vi "Use FGV3.vi"() -> ()   [LabVIEW 2022 SP3]
panel:
  in  "Publsher":dbl
  in  "stop":bool
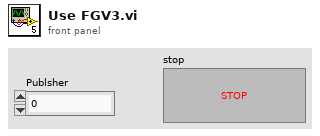
[diagram p1: front panel]
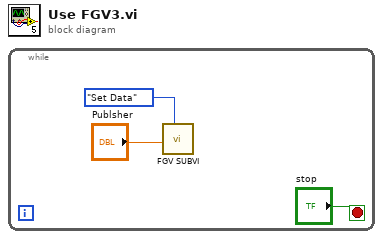
[diagram p0: block diagram]
diagram:
  n1 = while {
    stop <- "stop" stop-if-true
    n2 = call "FGV SUBVI.vi"("Enum"=enum16{"Get Data", "Set Data"}."Set Data", "Data Input in"="Publsher") -> ()  [unwired: 9 in, 1 out]
  }
